vi "Update Sample History.vi"(9 "Ball?":bool=TRUE, 10 "R in":T1, 11 "Sample":T1) -> (2 "covariance matrix V":T1, 3 "R out":T1, 5 "Sample Unwrapped":T1)   [LabVIEW 2017]
uses:
  <vilib>/Analysis/Matrix/Datatypes/RealMatrix.ctl
  <vilib>/Analysis/Matrix/Numeric/Multiply/Multiply - RM,R.vi
  <vilib>/gmath/NI_Gmath.lvlib
  <vilib>/Analysis/Matrix/NI_Matrix.lvlib
  <vilib>/Analysis/NI_AALPro.lvlib
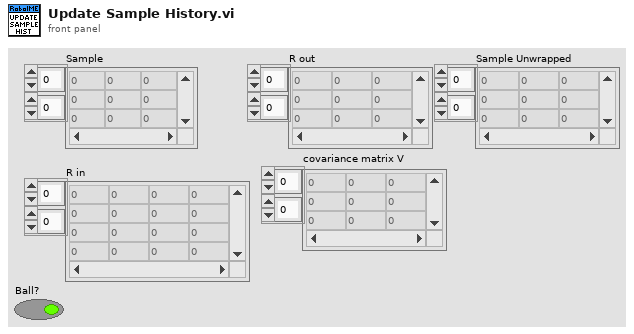
[diagram p1: front panel]
types:
  T1 = typedef "NI_Matrix.lvlib/RealMatrix.ctl" = dbl[][]
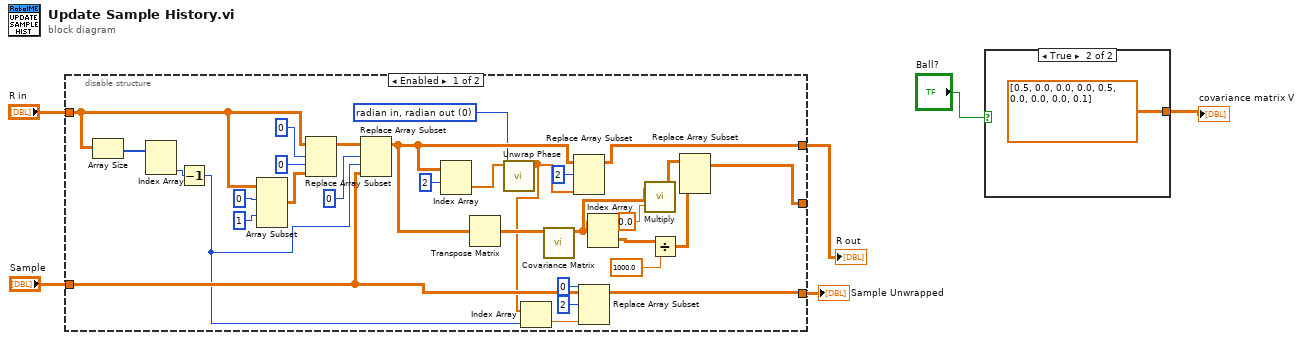
[diagram p0: block diagram]
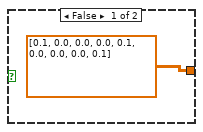
[diagram p2: hidden frame]
diagram:
  n1 = disable-structure shown="Enabled" {
    disable-tunnel: "Sample" -> [w18 _]
    disable-tunnel: "R in" -> [w21 w38]
    disable-tunnel: [w23 w38] -> w4
    disable-tunnel: [w12 _] -> w3
    disable-tunnel: [w7 _] -> _
    frame Enabled {
      w22 = 0 items=["radian in, radian out", "radian in, degree out", "degree in, degree out", "degree in, radian out"] ("phase unit")
      n2 = Array Size(array=w21) -> (size(s)=w20:i32[])
      n3 = Index Array(array=w20) -> (element #2=w19:i32)  [unwired: 2 in, 1 out]
      n4 = Decrement(x=w19) -> (x-1=w16:i32)
      n5 = Array Subset(array=w21, index (row)=0 ("index"), index (col)=1 ("index")) -> (w34:T1)  [unwired: 2 in]
      n6 = Replace Array Subset(array=w21, new element=w34, index (row)=0 ("disabled index (row)"), index (col)=0 ("disabled index (col)")) -> (w37:T1)
      n7 = Replace Array Subset(array=w37, new element=w18, index (row)=0, index (col)=w16) -> (w25:T1)
      n8 = Index Array(array=w25, index (row)=2) -> (element=w26:dbl[])  [unwired: 1 in]
      n9 = Transpose Matrix(1:w25) -> (0:w30:T1)
      n10 = call <vilib>:"Unwrap Phase.vi"("phase unit"=w22, "Phase"=w26) -> ("Unwrapped Phase"=w17:dbl[])  [unwired: 8 in, 1 out]
      n11 = Index Array(array=w17, index=w16) -> (element=w14:dbl)
      n12 = call <vilib>:"Covariance Matrix.vi"("X"=w30) -> ("covariance matrix V"=w11:T1)  [unwired: 9 in, 1 out]
      n13 = Replace Array Subset(array=w25, new element=w17, index (row)=2) -> (w23:T1)  [unwired: 1 in]
      n14 = Replace Array Subset(array=w18, new element=w14, index (row)=2, index (col)=0 ("disabled index (col)")) -> (w12:T1)
      n15 = Index Array(array=w11) -> (element=w28:T1)  [unwired: 2 in]
      n16 = call-poly <vilib>:"Multiply.vi"("Real Scalar c"=0.0 ("Real Matrix B"), "Real Matrix A"=w11) -> ("A * c"=w9:T1)
      n17 = Divide(x=w28, y=1000.0) -> (x/y=w8:T1)
      n18 = Replace Array Subset(array=w9, new element=w8) -> (w7:T1)  [unwired: 2 in]
    }
    frame Disabled {
    }
  }
  "R out" <- w4
  "Sample Unwrapped" <- w3
  n19 = case shown="True" "Ball?" {
    tunnel: [T1 [[0.1, 0.0, 0.0], [0.0, 0.1, 0.0], [0.0, 0.0, 0.1]] ("matrix") T1 [[0.5, 0.0, 0.0], [0.0, 0.5, 0.0], [0.0, 0.0, 0.1]] ("matrix")] -> w2
    frame False {
    }
    frame True {
    }
  }
  "covariance matrix V" <- w2
